vi "lvssh2_session_callback_register_send_32.vi"(11 "send":refnum<vi>) -> (0 "error out":errorcluster, 2 "stop event":refnum<user-event>, 3 "user event":refnum<user-event>)   [LabVIEW 2017, in "libssh2.lvlib"]
uses:
  libssh2.lvlib
  lvssh2_session_callback_send_function_input_args_32.ctl
  lvssh2_session_callback_send_handler_32.vi
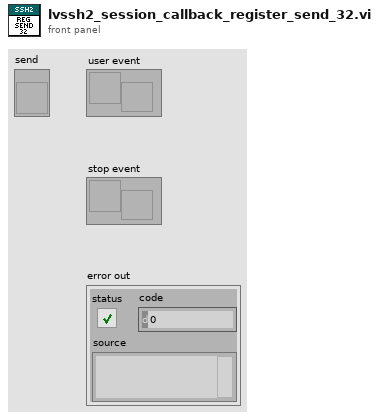
[diagram p1: front panel]
types:
  T1 = typedef "libssh2.lvlib/lvssh2_session_callback_send_function_input_args_32.ctl" = cluster{"*socket":u32, "buffer":u8[], "flags":i32, "*bytes_send":u32, "completion":u32}
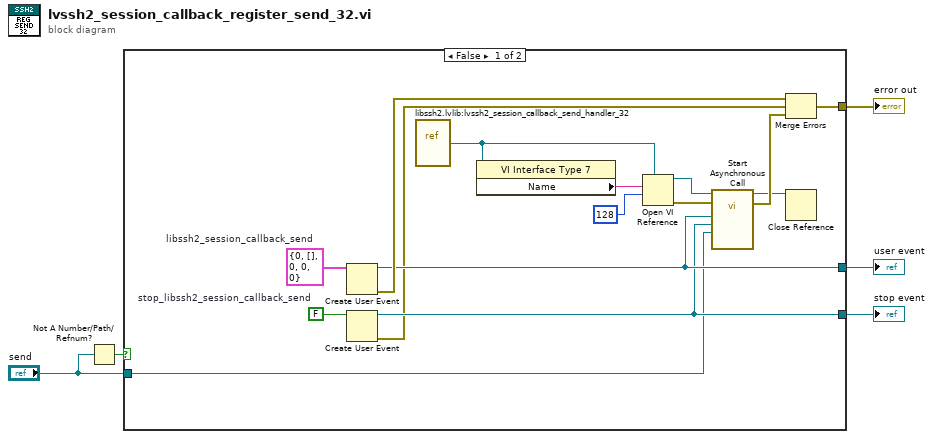
[diagram p0: block diagram]
diagram:
  n1 = Not A Number/Path/Refnum?(number/path/refnum="send") -> (NaN/Path/Refnum?=w2:bool)
  n2 = case shown="False" w2 {
    tunnel: [w11 _] -> w5
    tunnel: [w20 _] -> w4
    tunnel: "send" -> [w7 _]
    tunnel: [w10 _] -> w1
    frame False {
      w13 = FALSE  # stop_libssh2_session_callback_send
      w19 = T1 {"*socket"=0, "buffer"=[], "flags"=0, "*bytes_send"=0, "completion"=0}  # libssh2_session_callback_send
      n3 = Create User Event(user event datatype=w19) -> (user event=w11:refnum<user-event>, error out=w18:errorcluster)  [unwired: 1 in]
      n4 = Create User Event(user event datatype=w13) -> (user event=w10:refnum<user-event>, error out=w9:errorcluster)  [unwired: 1 in]
      n5 = vi-ref "libssh2.lvlib:lvssh2_session_callback_send_handler_32.vi"() -> ("vi reference"=w12:refnum<vi>)
      n6 = property class="VI Interface Type 7"(reference=w12) -> ("Name"=w17:string)  [unwired: 1 in, 2 out]
      n7 = Open VI Reference(type specifier VI Refnum (for type only)=w12, vi path=w17, options=128) -> (vi reference=w15:refnum<vi>, error out=w16:errorcluster)  [unwired: 3 in]
      n8 = call-by-ref "Start Asynchronous Call"(reference=w15, error in=w16, "lvssh2_session_callback_send"=w7, "Stop Event Ref"=w10, "User Event Ref"=w11) -> (reference out=w6:refnum<vi>, error out=w8:errorcluster)  [unwired: 9 in]
      n9 = Merge Errors(w18, w9, w8) -> (w20:errorcluster)
      n10 = Close Reference(reference=w6) -> ()  [unwired: 1 in, 1 out]
    }
    frame True {
    }
  }
  "user event" <- w5
  "error out" <- w4
  "stop event" <- w1
